vi "Get ControlRef from LibraryItem.vi"(8 "error in (no error)":errorcluster, 10 "Control Name":string, 11 "Library item in":refnum<vi>) -> (0 "error out":errorcluster, 1 "Control ref out":refnum<vi>, 2 "VI ref out":refnum<vi>, 3 "Library item out":refnum<vi>, 4 "Found?":bool)   [LabVIEW 2019, in "gRPC Template Creation Utility.lvlib"]
uses:
  gRPC Template Creation Utility.lvlib
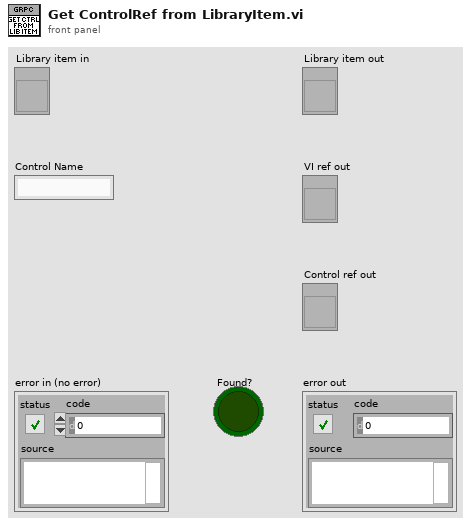
[diagram p1: front panel]
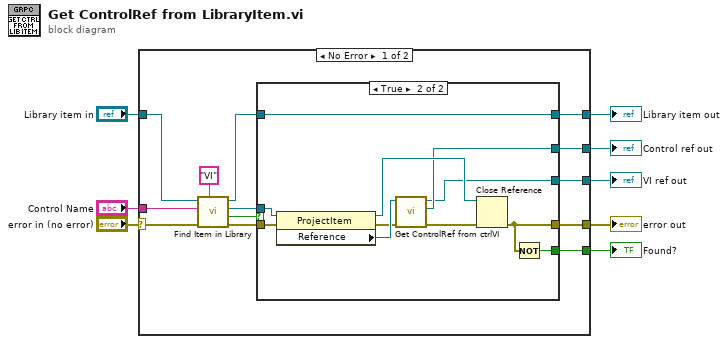
[diagram p0: block diagram]
diagram:
  n1 = case shown="No Error" "error in (no error)" {
    selector: "error in (no error)" -> [w12 w36]
    tunnel: [w21 _] -> w8
    tunnel: [w16 w36] -> w7
    tunnel: "Library item in" -> [w19 w35]
    tunnel: "Control Name" -> [w18 _]
    tunnel: [w13 w35] -> w3
    tunnel: [w10 _] -> w2
    tunnel: [w9 _] -> w1
    frame No Error {
      n2 = call "Find Item in Library.vi"("Item Type"="VI" ("Type"), "error in (no error)"=w12, "Item Name"=w18, "Library item in"=w19) -> ("error out"=w11:errorcluster, "Found?"=w15:bool, "Project Item (Library Item)"=w17:refnum<vi>, "Library item out"=w14:refnum<vi>)  [unwired: 4 in]
      n3 = case shown="True" w15 {
        tunnel: [_ w26] -> w21
        tunnel: w11 -> [w22 w32]
        tunnel: w17 -> [_ w31]
        tunnel: [w22 w28] -> w16
        tunnel: w14 -> [w23 w29]
        tunnel: [w23 w29] -> w13
        tunnel: [_ w27] -> w10
        tunnel: [_ w24] -> w9
        frame False {
        }
        frame True {
          n4 = property class="ProjectItem"(reference=w31, error in=w32) -> (reference out=w30:refnum<vi>, error out=w33:errorcluster, "Reference"=w34:refnum<vi>)
          n5 = call "Get ControlRef from ctrlVI.vi"("error in (no error)"=w33, "VI ref in"=w34) -> ("error out"=w25:errorcluster, "Control ref out"=w26:refnum<vi>, "VI ref out"=w24:refnum<vi>)  [unwired: 7 in]
          n6 = Close Reference(reference=w30, error in (no error)=w25) -> (error out=w28:errorcluster)
          n7 = Not(x=w28) -> (.not. x?=w27:bool)
        }
      }
    }
    frame Error {
    }
  }
  "Control ref out" <- w8
  "error out" <- w7
  "Library item out" <- w3
  "Found?" <- w2
  "VI ref out" <- w1
